vi "Get DI Status - Single.vi"(0 "reference in":refnum<class "DI.lvclass">, 2 "DI Channel Number (Zero Based)":i32, 5 "error in (no error)":errorcluster) -> (14 "reference out":refnum<class "DI.lvclass">, 15 "DI Channel Number (Zero Based) OUT":i32, 16 "DI Channel Status":bool, 19 "error out":errorcluster)   [LabVIEW 2017, in "DI.lvclass"]
uses:
  DI.lvclass
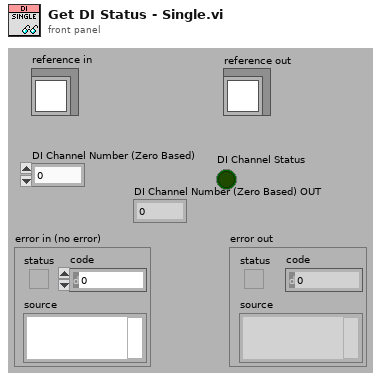
[diagram p1: front panel]
types:
  T1 = typedef "DI.lvclass/ObjectAttributes.ctl" = cluster{"DI Task":refnum<k21>, "DI Status":bool[], "DI Module Names (NI-Max Name)":string[], "Number of Channels Per DI Module":i32[], "Number of DI Modules":u32, "Number of Total DI Channels":u32, "DI On/Off Status":bool, "DO VI Reference":refnum<vi>}
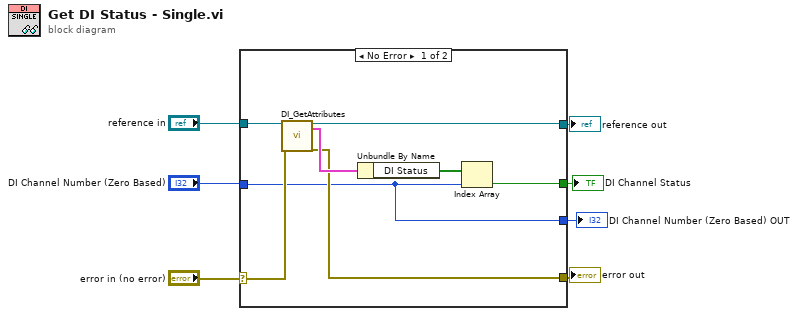
[diagram p0: block diagram]
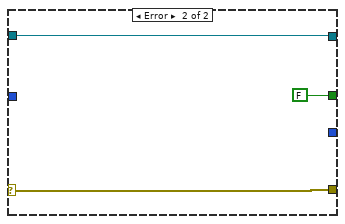
[diagram p2: hidden frame]
diagram:
  n1 = case shown="No Error" "error in (no error)" {
    selector: "error in (no error)" -> [w14 w18]
    tunnel: [w9 w18] -> w6
    tunnel: [w13 w17] -> w4
    tunnel: "reference in" -> [w15 w17]
    tunnel: "DI Channel Number (Zero Based)" -> [w8 _]
    tunnel: [w10 FALSE] -> w3
    tunnel: [w8 _] -> w1
    frame No Error {
      n2 = call "DI_GetAttributes.vi"("reference in"=w15, "error in (no error)"=w14) -> ("reference out"=w13:refnum<class "DI.lvclass">, "Data"=w11:T1, "error out"=w9:errorcluster)  [unwired: 14 in, 1 out]
      n3 = Unbundle By Name(w11) -> ("DI Status"=w12:bool[])
      n4 = Index Array(array=w12, index=w8) -> (element=w10:bool)
    }
    frame Error {
    }
  }
  "error out" <- w6
  "reference out" <- w4
  "DI Channel Status" <- w3
  "DI Channel Number (Zero Based) OUT" <- w1
